vi "Read step demand.vi"(11 "StepperMotor in":refnum<class "StepperMotor.lvclass">) -> (2 "step demand":i16=5000 min=10 max=5000, 3 "StepperMotor out":refnum<class "StepperMotor.lvclass">)   [LabVIEW 2013, in "StepperMotor.lvlib" / "StepperMotor.lvclass"]
uses:
  <userlib>/Common/Devices/StepperMotor/StepperMotor/StepperMotor.lvclass
  <userlib>/Common/Devices/StepperMotor/StepperMotor/StepperMotor.lvclass/StepperMotor.ctl
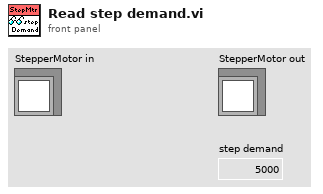
[diagram p1: front panel]
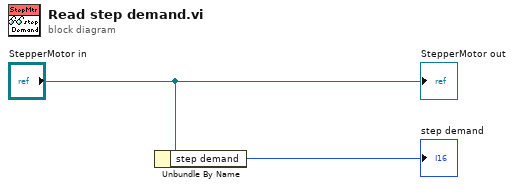
[diagram p0: block diagram]
diagram:
  n1 = Unbundle By Name("StepperMotor in") -> ("step demand"=→"step demand":i16)
  "StepperMotor out" <- "StepperMotor in"
